vi "Cycle 4 Main Spin Resume.vi"(0 "GEA2 Reference In":refnum<k24>, 1 "Basket Speeds (rpm)":u32[](array[numeric])=[125, 450, 700], 5 "GEA Inputs":T1={"Source"=228, "Destination"=35} {"Destination" format="%.0x"; "Source" format="%.0x"}, 7 "Standalone?":bool, 9 "Dwell Times (s)":dbl[](array[numeric])=[90.0, 30.0, 600.0], 11 "Error In":errorcluster, 12 "Basket Speed Tolerance (rpm)":u32=2) -> (4 "GEA2 Reference Out":refnum<k24>, 6 "Pass/Fail?":bool, 8 "Report Text":string, 15 "Error Out":errorcluster)   [LabVIEW 2016, in "TLMB.lvlib"]
uses:
  Projects/TLMB.lvlib
  Q:/Common/DLLs/GEA3/GeaCommunication.dll
  Common/DLLs/GEA3/GeaCommunication.dll
  Common/LabVIEW GEA2 Toolkit/LabVIEW_GEA2_Toolkit.lvlibp/type defs/Source_Destination.ctl
  Common/LabVIEW GEA2 Toolkit/LabVIEW_GEA2_Toolkit.lvlibp/type defs/ERD Read Data In.ctl
  Common/LabVIEW GEA2 Toolkit/LabVIEW_GEA2_Toolkit.lvlibp/type defs/Data Type.ctl
  TLMB Common/type defs/Drive Cycle Engine Request State.ctl
  Common/LabVIEW GEA2 Toolkit/LabVIEW_GEA2_Toolkit.lvlibp
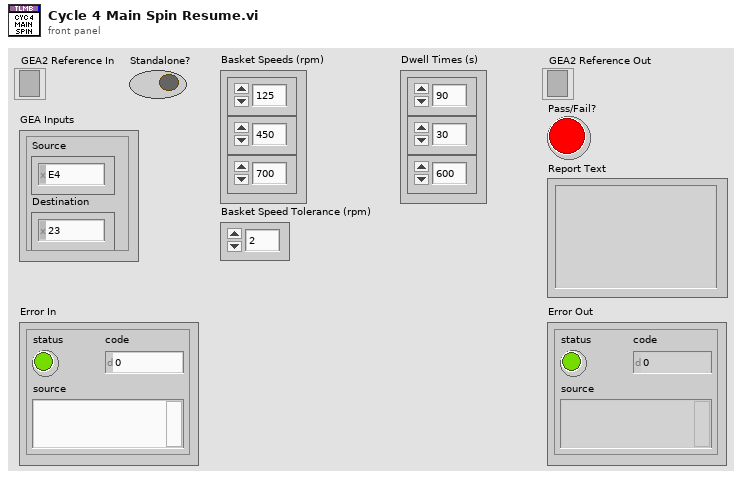
[diagram p1: front panel]
types:
  T1 = typedef "LabVIEW_GEA2_Toolkit.lvlibp/Source_Destination.ctl" = cluster{"Source":u8, "Destination":u8}
  T2 = typedef "LabVIEW_GEA2_Toolkit.lvlibp/ERD Read Data In.ctl" = cluster{"ERD Number":u16, "Data Type":T3}
  T3 = typedef "LabVIEW_GEA2_Toolkit.lvlibp/Data Type.ctl" = enum16{"string", "boolean", "uint8_t", "uint16_t", "uint32_t", "uint64_t", "int8_t", "int16_t", "int32_t", "int64_t"}
  T4 = typedef "TLMB.lvlib/Drive Cycle Engine Request State.ctl" = enum16{"Start", "Stop", "Pause", "Resume", "Select"}
  T5 = typedef "LabVIEW_GEA2_Toolkit.lvlibp/ERD Read Data Out.ctl" = cluster{"ERD Number":u16, "Data":string}
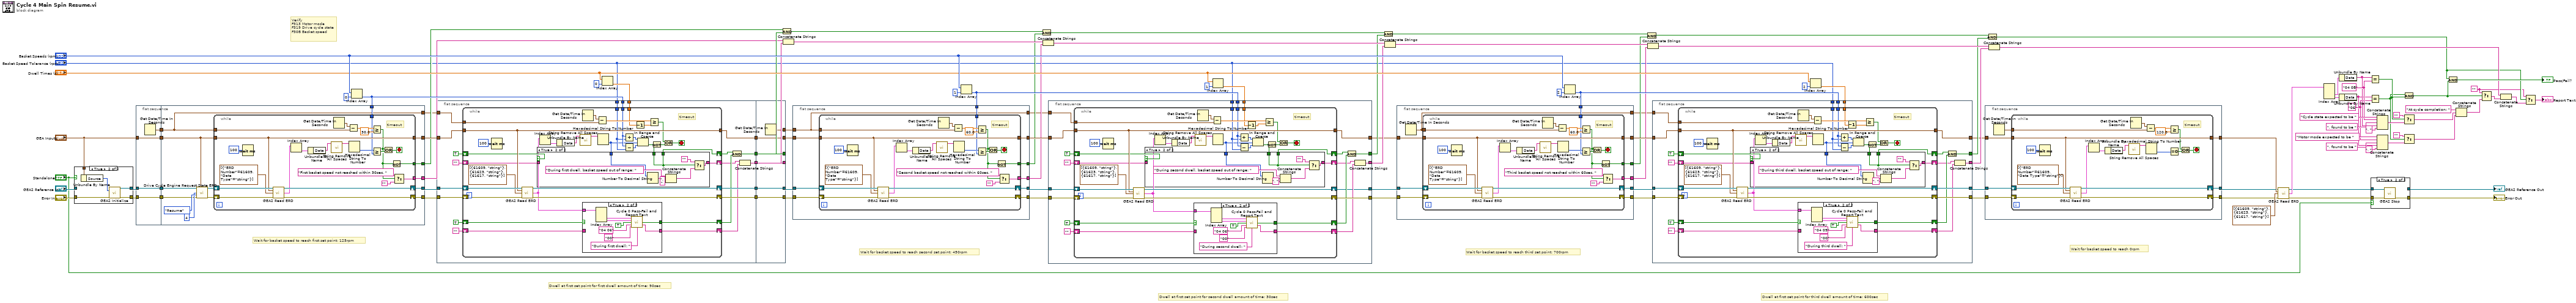
[diagram p0: block diagram]
diagram:
  w14 = ""
  w106 = "04 0B" ("y")
  w94 = "06" ("y")
  # "Wait for basket speed to reach 0rpm"
  # "Dwell at first set point for third dwell amount of time: 600sec"
  # "Wait for basket speed to reach third set point: 700rpm"
  # "Dwell at first set point for second dwell amount of time: 30sec"
  # "Wait for basket speed to reach second set point: 450rpm"
  # "Verify\nF313 Motor mode\nF319 Drive cycle state\nF30B Basket speed"
  # "Dwell at first set point for first dwell amount of time: 90sec"
  # "Wait for basket speed to reach first set point: 125rpm"
  n1 = case shown="True" "Standalone?" {
    tunnel: "GEA2 Reference In" -> [w113 _]
    tunnel: [w113 w118] -> w1
    tunnel: "Error In" -> [w112 w117]
    tunnel: [w112 w116] -> w2
    tunnel: "GEA Inputs" -> [_ w115]
    frame False {
    }
    frame True {
      n2 = Unbundle By Name(w115) -> ("Source"=w114:u8)
      n3 = call "GEA2 Initialize.vi"("Source Address"=w114, "error in"=w117) -> ("GEA2 Reference Out"=w118:refnum<k24>, "error out"=w116:errorcluster)  [unwired: 11 in, 1 out]
    }
  }
  n4 = flat-sequence {
    tunnel: "GEA Inputs" -> [w122]
    tunnel: [w122] -> w30
    tunnel: w2 -> [w119]
    tunnel: w1 -> [w120]
    tunnel: [w121] -> w29
    tunnel: [w120] -> w28
    tunnel: [w119] -> w27
    tunnel: [w136] -> w74
    tunnel: [w135] -> w75
    tunnel: [w134] -> w87
    tunnel: [w131] -> w53
    tunnel: [w132] -> w51
    tunnel: w56 -> [w133]
    tunnel: [w123] -> w33
    tunnel: w30 -> [w124]
    tunnel: w29 -> [w123]
    tunnel: w28 -> [w128]
    tunnel: w27 -> [w127]
    frame #0 {
      n5 = Get Date/Time In Seconds() -> (seconds since 1Jan1904=w121:timestamp)
    }
    frame #1 {
      n6 = call "Drive Cycle Engine Request State ERD.vi"("GEA2 Reference In"=w128, "GEA Inputs"=w124, "Cycle ID"=u8 4, "Drive Cycle Engine Request State"=Drive_Cycle_Engine_Request_State."Resume", "Error In"=w127) -> ("GEA2 Reference Out"=w126:refnum<k24>, "Error Out"=w125:errorcluster)  [unwired: 9 in]
      n7 = while {
        shift-right: [w159] -> w136
        shift-left: w125 -> [w160]
        shift-right: [w157] -> w135
        shift-left: w126 -> [w158]
        tunnel: w124 -> [w155]
        tunnel: [w155] -> w134
        tunnel: w123 -> [w137]
        tunnel: w133 -> [w145]
        tunnel: [w140] -> w132
        tunnel: [w138] -> w131
        stop <- w152 stop-if-true
        # "timeout"
        n8 = Wait (ms)(milliseconds to wait=u32 100) -> ()  [unwired: 1 out]
        n9 = call "GEA2 Read ERD.vi"("GEA2 Reference In"=w158, "GEA Inputs"=w155, "Read ERD List"=T2[] [{"ERD Number"=61609, "Data Type"=enum."string"}], "Error In"=w160) -> ("GEA2 Reference Out"=w157:refnum<k24>, "ERD Data Out"=w144:T5[], "Error Out"=w159:errorcluster)  [unwired: 8 in, 1 out]
        n10 = Index Array(array=w144) -> (element=w156:T5)  [unwired: 1 in]
        n11 = Unbundle By Name(w156) -> ("Data"=w148:string)
        n12 = call "String Remove All Spaces.vi"("Input String"=w148) -> ("Spaces Removed"=w149:string)  [unwired: 13 in, 1 out]
        n13 = Get Date/Time In Seconds() -> (seconds since 1Jan1904=w153:timestamp)
        n14 = Subtract(x=w153, y=w137) -> (x-y=w154:dbl)
        n15 = Hexadecimal String To Number(string=w149) -> (number=w147:u32)  [unwired: 2 in, 1 out]
        n16 = Greater Or Equal?(x=w154, y=30.0) -> (x >= y?=w139:bool)
        n17 = Greater Or Equal?(x=w147, y=w145) -> (x >= y?=w143:bool)
        n18 = Or(x=w139, y=w143) -> (x .or. y?=w152:bool)
        n19 = Not(x=w139) -> (.not. x?=w138:bool)
        n20 = Select(t="First basket speed not reached within 30sec. ", s=w139, f="") -> (s? t:f=w140:string)
      }
    }
  }
  n21 = Index Array(array="Basket Speeds (rpm)", index=0) -> (element=w56:u32)
  n22 = flat-sequence {
    tunnel: w77 -> [w173]
    tunnel: w56 -> [w172]
    tunnel: "Basket Speed Tolerance (rpm)" -> [w171]
    tunnel: w74 -> [w178]
    tunnel: w87 -> [w179]
    tunnel: w75 -> [w180]
    tunnel: w33 -> [w161]
    tunnel: [w176] -> w10
    tunnel: [w175] -> w9
    tunnel: [w174] -> w8
    tunnel: [w165] -> w7
    tunnel: [w162] -> w6
    tunnel: [w235] -> w11
    tunnel: [w236] -> w50
    tunnel: [w237] -> w52
    tunnel: [w238] -> w71
    tunnel: [w239] -> w73
    tunnel: [w240] -> w72
    tunnel: w10 -> [w240]
    tunnel: w9 -> [w239]
    tunnel: w8 -> [w238]
    tunnel: w7 -> [w237]
    tunnel: w6 -> [w236]
    frame #0 {
      n23 = while {
        shift-right: [w212] -> w176
        shift-left: w178 -> [w213]
        shift-right: [w210] -> w175
        shift-left: w180 -> [w211]
        tunnel: w179 -> [w208]
        tunnel: [w208] -> w174
        tunnel: w161 -> [w206]
        shift-right: [w190] -> w166
        shift-left: TRUE -> [w192]
        tunnel: w173 -> [w182]
        tunnel: w172 -> [w197]
        tunnel: w171 -> [w196]
        shift-right: [w194] -> w163
        shift-left: "" -> [w191]
        shift-right: [w184] -> w167
        shift-left: TRUE -> [w187]
        shift-right: [w185] -> w164
        shift-left: "" -> [w186]
        stop <- w204 stop-if-true
        # "timeout"
        n24 = Wait (ms)(milliseconds to wait=u32 100) -> ()  [unwired: 1 out]
        n25 = call "GEA2 Read ERD.vi"("GEA2 Reference In"=w211, "GEA Inputs"=w208, "Read ERD List"=T2[] [{"ERD Number"=61609, "Data Type"=enum."string"}, {"ERD Number"=61623, "Data Type"=enum."string"}, {"ERD Number"=61617, "Data Type"=enum."string"}], "Error In"=w213) -> ("GEA2 Reference Out"=w210:refnum<k24>, "ERD Data Out"=w183:T5[], "Error Out"=w212:errorcluster)  [unwired: 8 in, 1 out]
        n26 = Index Array(array=w183) -> (element=w209:T5)  [unwired: 1 in]
        n27 = Unbundle By Name(w209) -> ("Data"=w200:string)
        n28 = call "String Remove All Spaces.vi"("Input String"=w200) -> ("Spaces Removed"=w201:string)  [unwired: 13 in, 1 out]
        n29 = Get Date/Time In Seconds() -> (seconds since 1Jan1904=w205:timestamp)
        n30 = case shown="True" w187 {
          selector: w187 -> [w214 _]
          tunnel: w186 -> [w215 _]
          tunnel: [w215 w223] -> w185
          tunnel: [w214 w224] -> w184
          tunnel: w183 -> [_ w222]
          frame False {
          }
          frame True {
            n31 = Index Array(array=w222) -> (element #2=w220:T5, element #3=w219:T5)  [unwired: 3 in, 1 out]
            n32 = call "Cycle 0 Pass-Fail and Report Text.vi"("Drive Cycle State"=w220, "Motor Mode"=w219, "Previous Pass/Fail"=TRUE, "Cycle State Expected"="04 06", "Motor Mode Expected"="00", "Header"="During first dwell: ") -> ("Pass/Fail?"=w224:bool, "Report Text"=w223:string)  [unwired: 8 in]
          }
        }
        n33 = Subtract(x=w205, y=w206) -> (x-y=w207:dbl)
        n34 = Hexadecimal String To Number(string=w201) -> (number=w195:u32)  [unwired: 2 in, 1 out]
        n35 = Add(x=w197, y=w196) -> (x+y=w199:u32)
        n36 = Subtract(x=w197, y=w196) -> (x-y=w198:u32)
        n37 = Decrement(x=w182) -> (x-1=w181:dbl)
        n38 = In Range and Coerce(upper limit=w199, x=w195, lower limit=w198) -> (In Range?=w193:bool)  [unwired: 1 out]
        n39 = case shown="True" w192 {
          selector: w192 -> [w225 _]
          tunnel: w195 -> [_ w232]
          tunnel: [w226 w229] -> w194
          tunnel: w193 -> [_ w228]
          tunnel: w191 -> [w226 _]
          tunnel: [w225 w228] -> w190
          frame False {
          }
          frame True {
            n40 = Number To Decimal String(number=w232) -> (decimal integer string=w231:string)  [unwired: 1 in]
            n41 = Concatenate Strings("During first dwell, basket speed out of range: " ("string"), w231, ". " ("string")) -> (w230:string)
            n42 = Select(t="", s=w228, f=w230) -> (s? t:f=w229:string)
          }
        }
        n43 = Greater Or Equal?(x=w207, y=w181) -> (x >= y?=w188:bool)
        n44 = Not(x=w193) -> (.not. x?=w189:bool)
        n45 = Or(x=w188, y=w189) -> (x .or. y?=w204:bool)
      }
      n46 = And(x=w166, y=w167) -> (x .and. y?=w165:bool)
      n47 = Concatenate Strings(w163, w164) -> (w162:string)
    }
    frame #1 {
      n48 = Get Date/Time In Seconds() -> (seconds since 1Jan1904=w235:timestamp)
    }
  }
  n49 = Index Array(array="Dwell Times (s)", index=0) -> (element=w77:dbl)
  n50 = And(x=w53, y=w52) -> (x .and. y?=w49:bool)
  n51 = Concatenate Strings(w51, w50) -> (w48:string)
  n52 = flat-sequence {
    tunnel: [w247] -> w69
    tunnel: [w246] -> w68
    tunnel: [w245] -> w67
    tunnel: [w242] -> w46
    tunnel: [w243] -> w47
    tunnel: w66 -> [w244]
    tunnel: w72 -> [w248]
    tunnel: w71 -> [w249]
    tunnel: w73 -> [w250]
    tunnel: [w241] -> w32
    tunnel: w11 -> [w241]
    frame #0 {
      n53 = while {
        shift-right: [w273] -> w247
        shift-left: w248 -> [w274]
        shift-right: [w271] -> w246
        shift-left: w250 -> [w272]
        tunnel: w249 -> [w269]
        tunnel: [w269] -> w245
        tunnel: w241 -> [w251]
        tunnel: w244 -> [w259]
        tunnel: [w254] -> w243
        tunnel: [w252] -> w242
        stop <- w266 stop-if-true
        # "timeout"
        n54 = Wait (ms)(milliseconds to wait=u32 100) -> ()  [unwired: 1 out]
        n55 = call "GEA2 Read ERD.vi"("GEA2 Reference In"=w272, "GEA Inputs"=w269, "Read ERD List"=T2[] [{"ERD Number"=61609, "Data Type"=enum."string"}], "Error In"=w274) -> ("GEA2 Reference Out"=w271:refnum<k24>, "ERD Data Out"=w258:T5[], "Error Out"=w273:errorcluster)  [unwired: 8 in, 1 out]
        n56 = Index Array(array=w258) -> (element=w270:T5)  [unwired: 1 in]
        n57 = Unbundle By Name(w270) -> ("Data"=w262:string)
        n58 = call "String Remove All Spaces.vi"("Input String"=w262) -> ("Spaces Removed"=w263:string)  [unwired: 13 in, 1 out]
        n59 = Get Date/Time In Seconds() -> (seconds since 1Jan1904=w267:timestamp)
        n60 = Subtract(x=w267, y=w251) -> (x-y=w268:dbl)
        n61 = Hexadecimal String To Number(string=w263) -> (number=w261:u32)  [unwired: 2 in, 1 out]
        n62 = Greater Or Equal?(x=w268, y=60.0) -> (x >= y?=w253:bool)
        n63 = Greater Or Equal?(x=w261, y=w259) -> (x >= y?=w257:bool)
        n64 = Or(x=w253, y=w257) -> (x .or. y?=w266:bool)
        n65 = Not(x=w253) -> (.not. x?=w252:bool)
        n66 = Select(t="Second basket speed not reached within 60sec. ", s=w253, f="") -> (s? t:f=w254:string)
      }
    }
  }
  n67 = Index Array(array="Basket Speeds (rpm)", index=1) -> (element=w66:u32)
  n68 = And(x=w49, y=w46) -> (x .and. y?=w43:bool)
  n69 = Concatenate Strings(w48, w47) -> (w44:string)
  n70 = flat-sequence {
    tunnel: [w290] -> w3
    tunnel: [w289] -> w5
    tunnel: [w280] -> w42
    tunnel: [w277] -> w45
    tunnel: w64 -> [w288]
    tunnel: w66 -> [w287]
    tunnel: "Basket Speed Tolerance (rpm)" -> [w286]
    tunnel: w69 -> [w292]
    tunnel: w67 -> [w293]
    tunnel: w68 -> [w294]
    tunnel: [w276] -> w4
    tunnel: w32 -> [w275]
    frame #0 {
      n71 = while {
        shift-right: [w326] -> w290
        shift-left: w292 -> [w327]
        shift-right: [w324] -> w276
        shift-left: w294 -> [w325]
        tunnel: w293 -> [w322]
        tunnel: [w322] -> w289
        tunnel: w275 -> [w320]
        shift-right: [w304] -> w281
        shift-left: TRUE -> [w306]
        tunnel: w288 -> [w296]
        tunnel: w287 -> [w311]
        tunnel: w286 -> [w310]
        shift-right: [w308] -> w278
        shift-left: "" -> [w305]
        shift-right: [w298] -> w282
        shift-left: TRUE -> [w301]
        shift-right: [w299] -> w279
        shift-left: "" -> [w300]
        stop <- w318 stop-if-true
        # "timeout"
        n72 = Wait (ms)(milliseconds to wait=u32 100) -> ()  [unwired: 1 out]
        n73 = call "GEA2 Read ERD.vi"("GEA2 Reference In"=w325, "GEA Inputs"=w322, "Read ERD List"=T2[] [{"ERD Number"=61609, "Data Type"=enum."string"}, {"ERD Number"=61623, "Data Type"=enum."string"}, {"ERD Number"=61617, "Data Type"=enum."string"}], "Error In"=w327) -> ("GEA2 Reference Out"=w324:refnum<k24>, "ERD Data Out"=w297:T5[], "Error Out"=w326:errorcluster)  [unwired: 8 in, 1 out]
        n74 = Index Array(array=w297) -> (element=w323:T5)  [unwired: 1 in]
        n75 = Unbundle By Name(w323) -> ("Data"=w314:string)
        n76 = case shown="True" w301 {
          selector: w301 -> [w328 _]
          tunnel: w300 -> [w329 _]
          tunnel: [w329 w337] -> w299
          tunnel: [w328 w338] -> w298
          tunnel: w297 -> [_ w336]
          frame False {
          }
          frame True {
            n77 = Index Array(array=w336) -> (element #2=w334:T5, element #3=w333:T5)  [unwired: 3 in, 1 out]
            n78 = call "Cycle 0 Pass-Fail and Report Text.vi"("Drive Cycle State"=w334, "Motor Mode"=w333, "Previous Pass/Fail"=TRUE, "Cycle State Expected"="04 06", "Motor Mode Expected"="00", "Header"="During second dwell: ") -> ("Pass/Fail?"=w338:bool, "Report Text"=w337:string)  [unwired: 8 in]
          }
        }
        n79 = call "String Remove All Spaces.vi"("Input String"=w314) -> ("Spaces Removed"=w315:string)  [unwired: 13 in, 1 out]
        n80 = Get Date/Time In Seconds() -> (seconds since 1Jan1904=w319:timestamp)
        n81 = Subtract(x=w319, y=w320) -> (x-y=w321:dbl)
        n82 = Hexadecimal String To Number(string=w315) -> (number=w309:u32)  [unwired: 2 in, 1 out]
        n83 = Add(x=w311, y=w310) -> (x+y=w313:u32)
        n84 = Subtract(x=w311, y=w310) -> (x-y=w312:u32)
        n85 = Decrement(x=w296) -> (x-1=w295:dbl)
        n86 = In Range and Coerce(upper limit=w313, x=w309, lower limit=w312) -> (In Range?=w307:bool)  [unwired: 1 out]
        n87 = case shown="True" w306 {
          selector: w306 -> [w339 _]
          tunnel: w309 -> [_ w346]
          tunnel: [w340 w343] -> w308
          tunnel: w307 -> [_ w342]
          tunnel: w305 -> [w340 _]
          tunnel: [w339 w342] -> w304
          frame False {
          }
          frame True {
            n88 = Number To Decimal String(number=w346) -> (decimal integer string=w345:string)  [unwired: 1 in]
            n89 = Concatenate Strings("During second dwell, basket speed out of range: " ("string"), w345, ". " ("string")) -> (w344:string)
            n90 = Select(t="", s=w342, f=w344) -> (s? t:f=w343:string)
          }
        }
        n91 = Greater Or Equal?(x=w321, y=w295) -> (x >= y?=w302:bool)
        n92 = Not(x=w307) -> (.not. x?=w303:bool)
        n93 = Or(x=w302, y=w303) -> (x .or. y?=w318:bool)
      }
      n94 = And(x=w281, y=w282) -> (x .and. y?=w280:bool)
      n95 = Concatenate Strings(w278, w279) -> (w277:string)
    }
  }
  n96 = Index Array(array="Dwell Times (s)", index=1) -> (element=w64:dbl)
  n97 = And(x=w43, y=w42) -> (x .and. y?=w41:bool)
  n98 = Concatenate Strings(w44, w45) -> (w40:string)
  n99 = flat-sequence {
    tunnel: [w355] -> w62
    tunnel: [w354] -> w61
    tunnel: [w353] -> w60
    tunnel: [w350] -> w38
    tunnel: [w351] -> w39
    tunnel: w59 -> [w352]
    tunnel: w3 -> [w356]
    tunnel: w5 -> [w357]
    tunnel: w4 -> [w358]
    tunnel: [w349] -> w31
    frame #0 {
      n100 = Get Date/Time In Seconds() -> (seconds since 1Jan1904=w349:timestamp)
      n101 = while {
        shift-right: [w381] -> w355
        shift-left: w356 -> [w382]
        shift-right: [w379] -> w354
        shift-left: w358 -> [w380]
        tunnel: w357 -> [w377]
        tunnel: [w377] -> w353
        tunnel: w349 -> [w359]
        tunnel: w352 -> [w367]
        tunnel: [w362] -> w351
        tunnel: [w360] -> w350
        stop <- w374 stop-if-true
        # "timeout"
        n102 = Wait (ms)(milliseconds to wait=u32 100) -> ()  [unwired: 1 out]
        n103 = call "GEA2 Read ERD.vi"("GEA2 Reference In"=w380, "GEA Inputs"=w377, "Read ERD List"=T2[] [{"ERD Number"=61609, "Data Type"=enum."string"}], "Error In"=w382) -> ("GEA2 Reference Out"=w379:refnum<k24>, "ERD Data Out"=w366:T5[], "Error Out"=w381:errorcluster)  [unwired: 8 in, 1 out]
        n104 = Index Array(array=w366) -> (element=w378:T5)  [unwired: 1 in]
        n105 = Unbundle By Name(w378) -> ("Data"=w370:string)
        n106 = call "String Remove All Spaces.vi"("Input String"=w370) -> ("Spaces Removed"=w371:string)  [unwired: 13 in, 1 out]
        n107 = Get Date/Time In Seconds() -> (seconds since 1Jan1904=w375:timestamp)
        n108 = Subtract(x=w375, y=w359) -> (x-y=w376:dbl)
        n109 = Hexadecimal String To Number(string=w371) -> (number=w369:u32)  [unwired: 2 in, 1 out]
        n110 = Greater Or Equal?(x=w376, y=60.0) -> (x >= y?=w361:bool)
        n111 = Greater Or Equal?(x=w369, y=w367) -> (x >= y?=w365:bool)
        n112 = Or(x=w361, y=w365) -> (x .or. y?=w374:bool)
        n113 = Not(x=w361) -> (.not. x?=w360:bool)
        n114 = Select(t="Third basket speed not reached within 60sec. ", s=w361, f="") -> (s? t:f=w362:string)
      }
    }
  }
  n115 = Index Array(array="Basket Speeds (rpm)", index=2) -> (element=w59:u32)
  n116 = And(x=w41, y=w38) -> (x .and. y?=w37:bool)
  n117 = Concatenate Strings(w40, w39) -> (w36:string)
  n118 = flat-sequence {
    tunnel: [w398] -> w25
    tunnel: [w397] -> w26
    tunnel: [w396] -> w24
    tunnel: [w387] -> w34
    tunnel: [w384] -> w35
    tunnel: w57 -> [w395]
    tunnel: w59 -> [w394]
    tunnel: "Basket Speed Tolerance (rpm)" -> [w393]
    tunnel: w62 -> [w400]
    tunnel: w60 -> [w401]
    tunnel: w61 -> [w402]
    tunnel: w31 -> [w383]
    frame #0 {
      n119 = while {
        shift-right: [w434] -> w398
        shift-left: w400 -> [w435]
        shift-right: [w432] -> w397
        shift-left: w402 -> [w433]
        tunnel: w401 -> [w430]
        tunnel: [w430] -> w396
        tunnel: w383 -> [w428]
        shift-right: [w412] -> w388
        shift-left: TRUE -> [w414]
        tunnel: w395 -> [w404]
        tunnel: w394 -> [w419]
        tunnel: w393 -> [w418]
        shift-right: [w416] -> w385
        shift-left: "" -> [w413]
        shift-right: [w406] -> w389
        shift-left: TRUE -> [w409]
        shift-right: [w407] -> w386
        shift-left: "" -> [w408]
        stop <- w426 stop-if-true
        # "timeout"
        n120 = Wait (ms)(milliseconds to wait=u32 100) -> ()  [unwired: 1 out]
        n121 = call "GEA2 Read ERD.vi"("GEA2 Reference In"=w433, "GEA Inputs"=w430, "Read ERD List"=T2[] [{"ERD Number"=61609, "Data Type"=enum."string"}, {"ERD Number"=61623, "Data Type"=enum."string"}, {"ERD Number"=61617, "Data Type"=enum."string"}], "Error In"=w435) -> ("GEA2 Reference Out"=w432:refnum<k24>, "ERD Data Out"=w405:T5[], "Error Out"=w434:errorcluster)  [unwired: 8 in, 1 out]
        n122 = Index Array(array=w405) -> (element=w431:T5)  [unwired: 1 in]
        n123 = Unbundle By Name(w431) -> ("Data"=w422:string)
        n124 = call "String Remove All Spaces.vi"("Input String"=w422) -> ("Spaces Removed"=w423:string)  [unwired: 13 in, 1 out]
        n125 = Get Date/Time In Seconds() -> (seconds since 1Jan1904=w427:timestamp)
        n126 = case shown="True" w409 {
          selector: w409 -> [w436 _]
          tunnel: w408 -> [w437 _]
          tunnel: [w437 w445] -> w407
          tunnel: [w436 w446] -> w406
          tunnel: w405 -> [_ w444]
          frame False {
          }
          frame True {
            n127 = Index Array(array=w444) -> (element #2=w442:T5, element #3=w441:T5)  [unwired: 3 in, 1 out]
            n128 = call "Cycle 0 Pass-Fail and Report Text.vi"("Drive Cycle State"=w442, "Motor Mode"=w441, "Previous Pass/Fail"=TRUE, "Cycle State Expected"="04 09", "Motor Mode Expected"="00", "Header"="During third dwell: ") -> ("Pass/Fail?"=w446:bool, "Report Text"=w445:string)  [unwired: 8 in]
          }
        }
        n129 = Subtract(x=w427, y=w428) -> (x-y=w429:dbl)
        n130 = Hexadecimal String To Number(string=w423) -> (number=w417:u32)  [unwired: 2 in, 1 out]
        n131 = Add(x=w419, y=w418) -> (x+y=w421:u32)
        n132 = Subtract(x=w419, y=w418) -> (x-y=w420:u32)
        n133 = Decrement(x=w404) -> (x-1=w403:dbl)
        n134 = In Range and Coerce(upper limit=w421, x=w417, lower limit=w420) -> (In Range?=w415:bool)  [unwired: 1 out]
        n135 = case shown="True" w414 {
          selector: w414 -> [w447 _]
          tunnel: w417 -> [_ w454]
          tunnel: [w448 w451] -> w416
          tunnel: w415 -> [_ w450]
          tunnel: w413 -> [w448 _]
          tunnel: [w447 w450] -> w412
          frame False {
          }
          frame True {
            n136 = Number To Decimal String(number=w454) -> (decimal integer string=w453:string)  [unwired: 1 in]
            n137 = Concatenate Strings("During third dwell, basket speed out of range: " ("string"), w453, ". " ("string")) -> (w452:string)
            n138 = Select(t="", s=w450, f=w452) -> (s? t:f=w451:string)
          }
        }
        n139 = Greater Or Equal?(x=w429, y=w403) -> (x >= y?=w410:bool)
        n140 = Not(x=w415) -> (.not. x?=w411:bool)
        n141 = Or(x=w410, y=w411) -> (x .or. y?=w426:bool)
      }
      n142 = And(x=w388, y=w389) -> (x .and. y?=w387:bool)
      n143 = Concatenate Strings(w385, w386) -> (w384:string)
    }
  }
  n144 = Index Array(array="Dwell Times (s)", index=2) -> (element=w57:dbl)
  n145 = flat-sequence {
    tunnel: [w459] -> w21
    tunnel: [w458] -> w22
    tunnel: [w457] -> w23
    tunnel: w25 -> [w461]
    tunnel: w24 -> [w462]
    tunnel: w26 -> [w463]
    frame #0 {
      n146 = Get Date/Time In Seconds() -> (seconds since 1Jan1904=w460:timestamp)
      n147 = while {
        shift-right: [w481] -> w459
        shift-left: w461 -> [w482]
        shift-right: [w479] -> w458
        shift-left: w463 -> [w480]
        tunnel: w462 -> [w477]
        tunnel: [w477] -> w457
        tunnel: w460 -> [w464]
        stop <- w474 stop-if-true
        # "timeout"
        n148 = Wait (ms)(milliseconds to wait=u32 100) -> ()  [unwired: 1 out]
        n149 = call "GEA2 Read ERD.vi"("GEA2 Reference In"=w480, "GEA Inputs"=w477, "Read ERD List"=T2[] [{"ERD Number"=61609, "Data Type"=enum."string"}], "Error In"=w482) -> ("GEA2 Reference Out"=w479:refnum<k24>, "ERD Data Out"=w467:T5[], "Error Out"=w481:errorcluster)  [unwired: 8 in, 1 out]
        n150 = Index Array(array=w467) -> (element=w478:T5)  [unwired: 1 in]
        n151 = Unbundle By Name(w478) -> ("Data"=w470:string)
        n152 = call "String Remove All Spaces.vi"("Input String"=w470) -> ("Spaces Removed"=w471:string)  [unwired: 13 in, 1 out]
        n153 = Get Date/Time In Seconds() -> (seconds since 1Jan1904=w475:timestamp)
        n154 = Subtract(x=w475, y=w464) -> (x-y=w476:dbl)
        n155 = Hexadecimal String To Number(string=w471) -> (number=w469:u32)  [unwired: 2 in, 1 out]
        n156 = Greater Or Equal?(x=w476, y=120.0) -> (x >= y?=w465:bool)
        n157 = Equal To 0?(x=w469) -> (x = 0?=w466:bool)
        n158 = Or(x=w465, y=w466) -> (x .or. y?=w474:bool)
      }
    }
  }
  n159 = And(x=w37, y=w34) -> (x .and. y?=w15:bool)
  n160 = Concatenate Strings(w36, w35) -> (w17:string)
  n161 = call "GEA2 Read ERD.vi"("GEA2 Reference In"=w22, "GEA Inputs"=w23, "Read ERD List"=T2[] [{"ERD Number"=61609, "Data Type"=enum."string"}, {"ERD Number"=61623, "Data Type"=enum."string"}, {"ERD Number"=61617, "Data Type"=enum."string"}], "Error In"=w21) -> ("GEA2 Reference Out"=w81:refnum<k24>, "ERD Data Out"=w108:T5[], "Error Out"=w83:errorcluster)  [unwired: 8 in, 1 out]
  n162 = Index Array(array=w108) -> (element #2=w111:T5, element #3=w110:T5)  [unwired: 3 in, 1 out]
  n163 = Unbundle By Name(w111) -> ("Data"=w104:string)
  n164 = Unbundle By Name(w110) -> ("Data"=w92:string)
  n165 = Equal?(x=w104, y=w106) -> (x = y?=w101:bool)
  n166 = Equal?(x=w92, y=w94) -> (x = y?=w100:bool)
  n167 = case shown="True" "Standalone?" {
    tunnel: [w483 w487] -> w84
    tunnel: w83 -> [w483 w486]
    tunnel: w81 -> [w484 w485]
    tunnel: [w484 _] -> w80
    frame False {
    }
    frame True {
      n168 = call "GEA2 Stop.vi"("GEA2 Reference In"=w485, "Error In"=w486) -> ("Error Out"=w487:errorcluster)  [unwired: 13 in]
    }
  }
  "GEA2 Reference Out" <- w80
  "Error Out" <- w84
  n169 = Concatenate Strings("Cycle state expected to be " ("string"), w106, ", found to be " ("string"), w104, ". " ("string")) -> (w102:string)
  n170 = Concatenate Strings("Motor mode expected to be " ("string"), w94, ", found to be " ("string"), w92, ". " ("string")) -> (w97:string)
  n171 = And(x=w100, y=w101) -> (x .and. y?=w19:bool)
  n172 = Select(t="", s=w101, f=w102) -> (s? t:f=w90:string)
  n173 = Select(t="", s=w100, f=w97) -> (s? t:f=w89:string)
  n174 = And(x=w15, y=w19) -> (x .and. y?=→"Pass/Fail?":bool)
  n175 = Concatenate Strings("At cycle completion: " ("string"), w90, w89) -> (w96:string)
  n176 = Select(t=w14, s=w19, f=w96) -> (s? t:f=w16:string)
  n177 = Concatenate Strings(w17, w16) -> (w13:string)
  n178 = Select(t=w14, s=w15, f=w13) -> (s? t:f=→"Report Text":string)
